vi "Measurement UI.vi"() -> ()   [LabVIEW 2020, in "Line Regulation.lvlib"]
uses:
  Line Regulation.lvlib
panel:
  out "Test Results.Input Voltage in V":dbl[](array[numeric])
  out "Output Voltage in V":dbl[](array[numeric])
  in  "Load SMU":refnum<k15>="DPS_4145_1/3"
  in  "Load DMM":refnum<k15>="DMM2"
  in  "Input DMM":refnum<k15>="DMM1"
  in  "Input SMU":refnum<k15>="DPS_4145_1/1"
  in  "Step":dbl=0.01
  in  "Stop":dbl=0.43
  in  "Start":dbl=0.03
  out "Line Regulation":cluster{"Iload (mA)":dbl[], "Vout (V)":dbl[]}(graph)
  out "Line Regulation (%)":dbl format="%#.3g"
  out "Line Regulation (%/V)":dbl format="%#.3g"
  in  "Nominal Output Voltage in V":dbl=3.3
  in  "Load Current in A":dbl=0.005
  # "Measurement Configurations"
  # "Measurement Results"
  # "Instruments"
  # "Input Voltage in V"
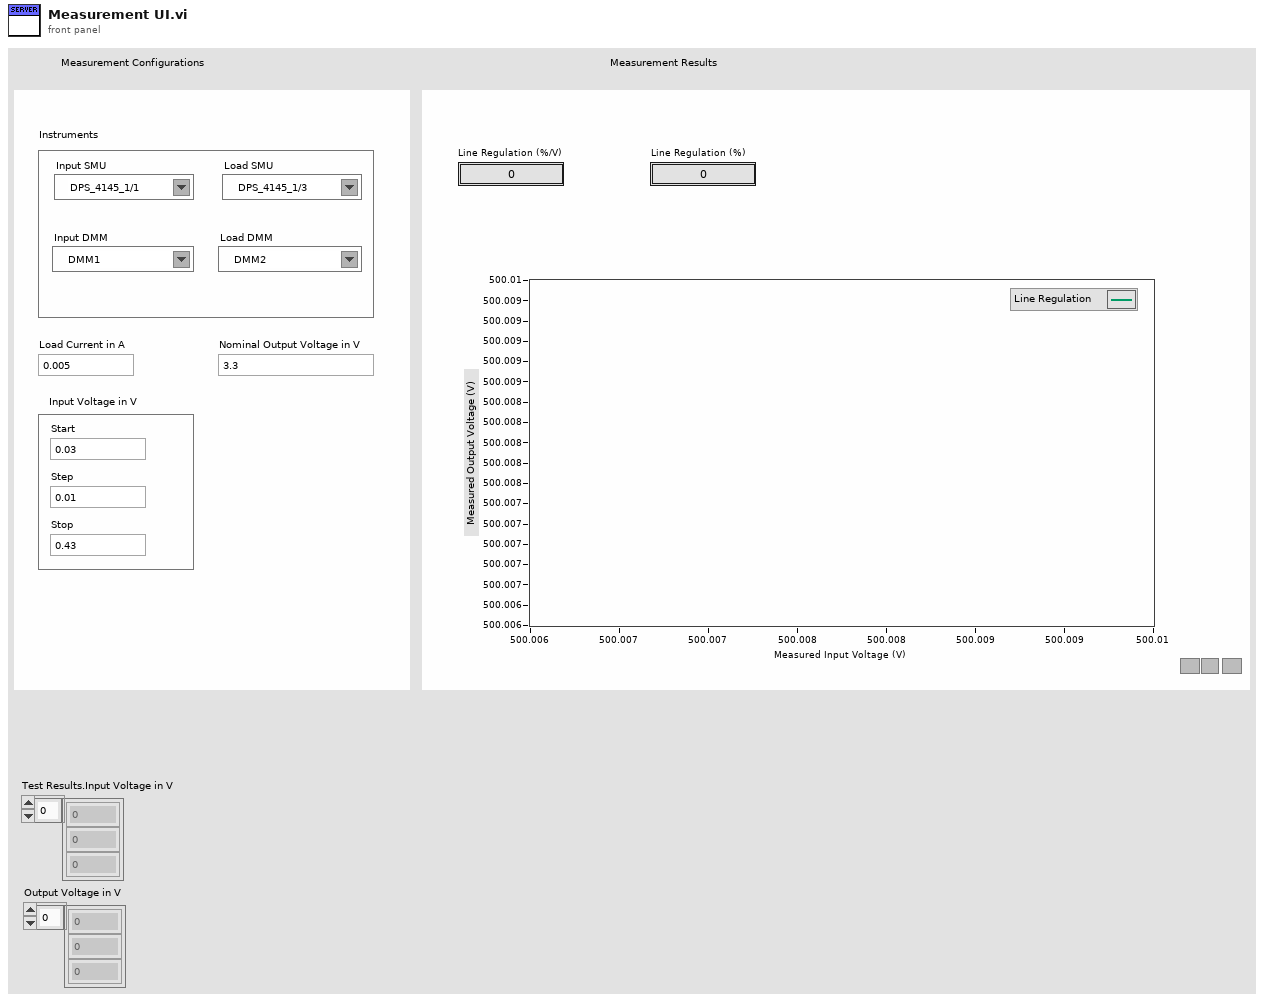
[diagram p1: front panel]
types:
  T1 = cluster{"Test Results.Input Voltage in V":dbl[], "Output Voltage in V":dbl[]}
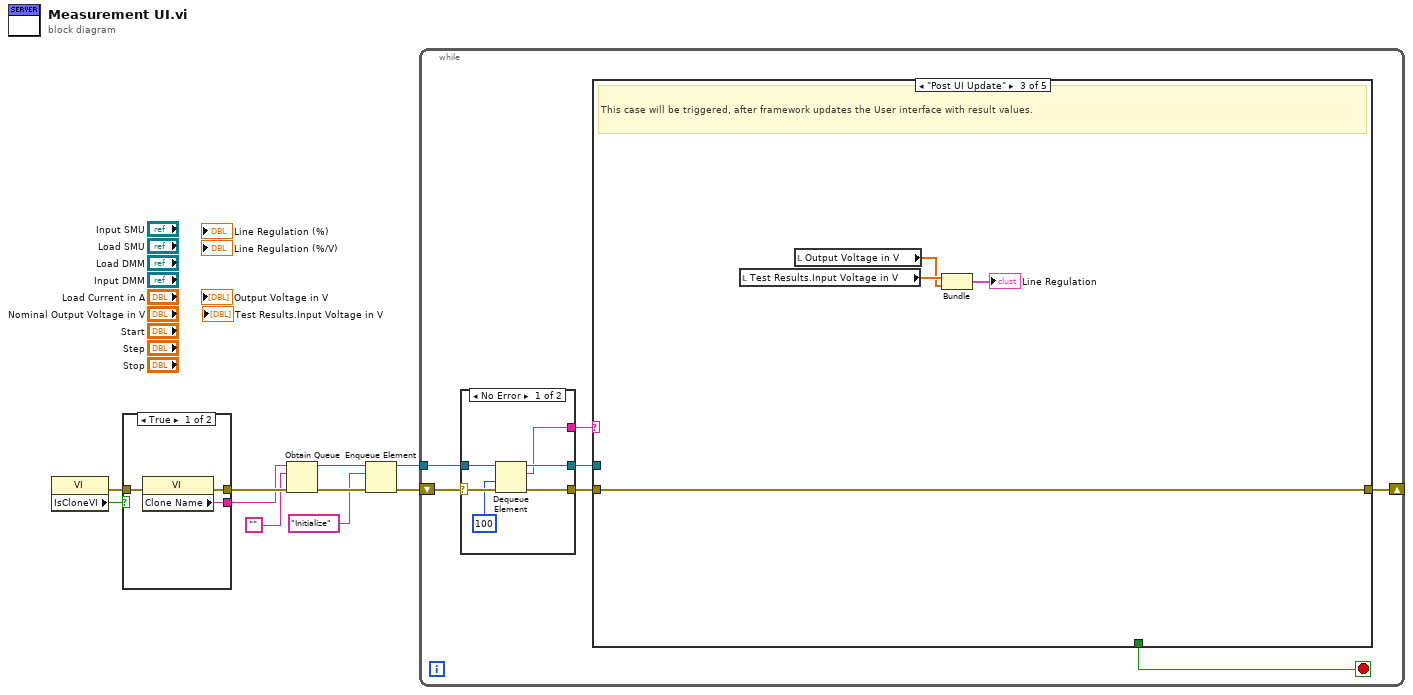
[diagram p0: block diagram]
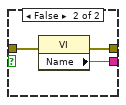
[diagram p2: hidden frame]
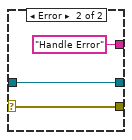
[diagram p3: hidden frame]
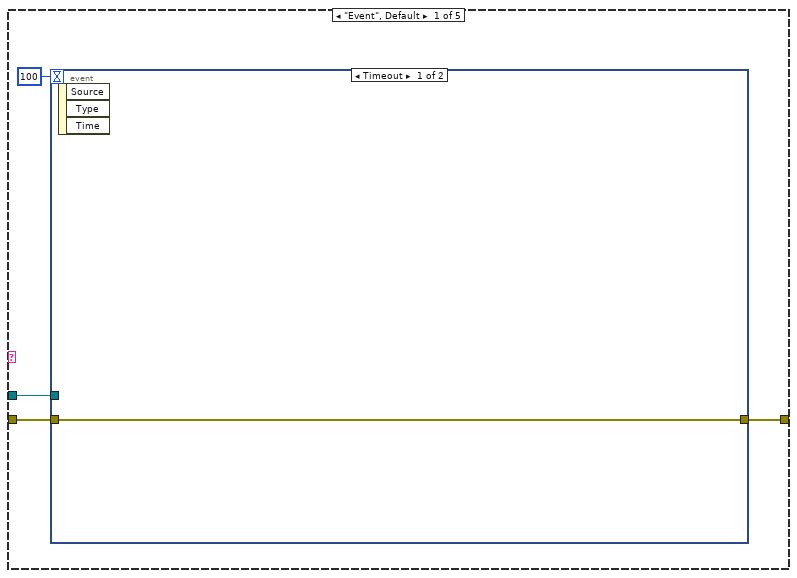
[diagram p4: hidden frame]
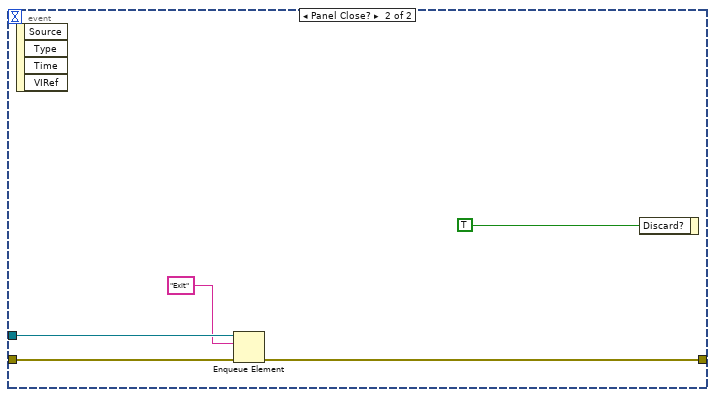
[diagram p5: hidden frame]
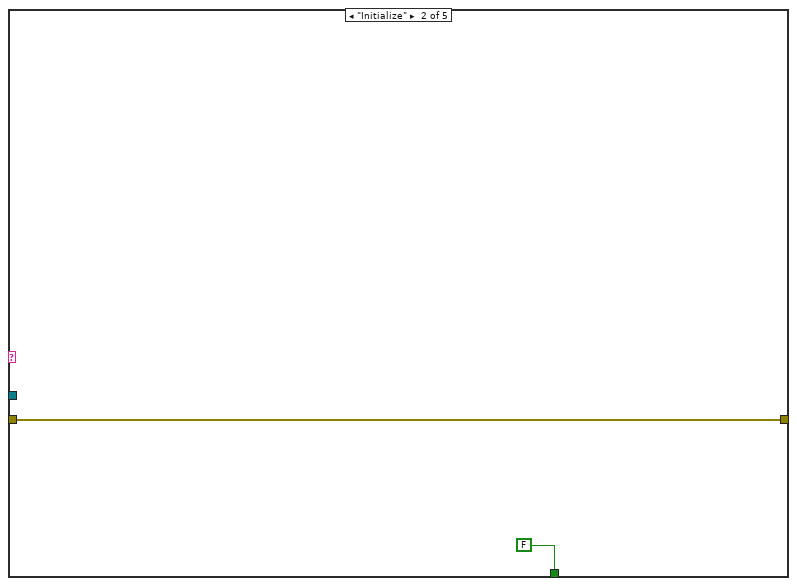
[diagram p6: hidden frame]
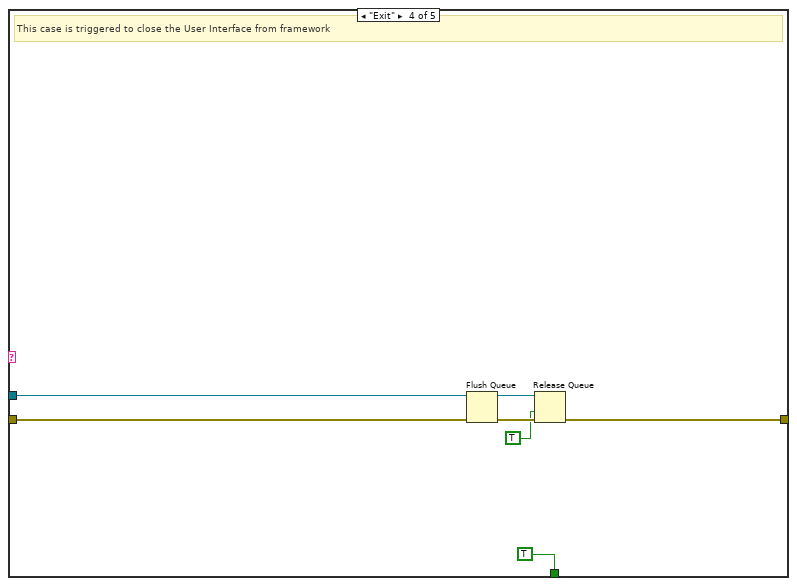
[diagram p7: hidden frame]
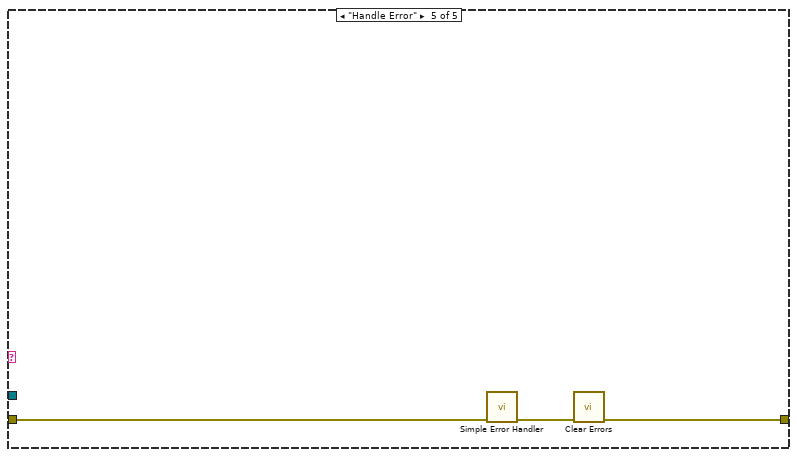
[diagram p8: hidden frame]
diagram:
  n1 = property class="VI"() -> (error out=w1:errorcluster, "IsCloneVI"=w2:bool)  [unwired: 2 in, 1 out]
  n2 = case shown="True" w2 {
    tunnel: [w13 w16] -> w10
    tunnel: [w12 w15] -> w9
    tunnel: w1 -> [w11 w14]
    frame True {
      n3 = property class="VI"(error in=w11) -> (error out=w13:errorcluster, "Clone Name"=w12:string)  [unwired: 1 in, 1 out]
    }
    frame False {
      n4 = property class="VI"(error in=w14) -> (error out=w16:errorcluster, "Name"=w15:string)  [unwired: 1 in, 1 out]
    }
  }
  n5 = Obtain Queue(name (unnamed)=w9, element data type="", error in (no error)=w10) -> (queue out=w6:refnum<queue>, error out=w8:errorcluster)  [unwired: 2 in, 1 out]
  n6 = Enqueue Element(queue=w6, element="Initialize", error in (no error)=w8) -> (queue out=w5:refnum<queue>, error out=w7:errorcluster)  [unwired: 1 in, 1 out]
  n7 = while {
    shift-right: [w18] -> _
    shift-left: w7 -> [w23]
    tunnel: w5 -> [w21]
    stop <- w17 stop-if-true
    n8 = case shown="No Error" w23 {
      selector: w23 -> [w29 w32]
      tunnel: [w28 w32] -> w22
      tunnel: w21 -> [w27 w31]
      tunnel: [w26 w31] -> w20
      tunnel: [w25 "Handle Error"] -> w19
      frame No Error {
        n9 = Dequeue Element(queue=w27, timeout in ms (-1)=100, error in (no error)=w29) -> (queue out=w26:refnum<queue>, element=w25:string, error out=w28:errorcluster)  [unwired: 1 out]
      }
      frame Error {
      }
    }
    n10 = case shown="\"Post UI Update\"" w19 {
      tunnel: w22 -> [w35 w44 w48 w55 w58]
      tunnel: w20 -> [w33 _ _ w53 _]
      tunnel: [w36 w44 w48 w50 w56] -> w18
      tunnel: [_ FALSE _ TRUE _] -> w17
      frame "Event", Default {
        n11 = event shown="[0] Timeout" {
          selector: _ -> [_ _]
          dyn-events: _ -> [_ _]
          timeout: 100 -> [_ _]
          tunnel: [w37 w40] -> w36
          tunnel: w35 -> [w37 w41]
          tunnel: w33 -> [_ w39]
          event Timeout {
            n12 = event-data() -> ()  [unwired: 1 in, 3 out]
          }
          event Panel Close? {
            n13 = event-data() -> ()  [unwired: 1 in, 4 out]
            n14 = Enqueue Element(queue=w39, element="Exit", error in (no error)=w41) -> (error out=w40:errorcluster)  [unwired: 1 in, 2 out]
            n15 = event-data("Discard?"=TRUE) -> ()  [unwired: 1 in, 1 out]
          }
        }
      }
      frame "Initialize" {
      }
      frame "Post UI Update" {
        # "This case will be triggered, after framework updates the User interface with result values."
        n16 = local read "Test Results.Input Voltage in V"() -> (w47:dbl[])
        n17 = local read "Output Voltage in V"() -> (w46:dbl[])
        n18 = Bundle("Test Results.Input Voltage in V"=w47, "Output Voltage in V"=w46) -> (→"Line Regulation":T1)  [unwired: 1 in]
      }
      frame "Exit" {
        # "This case is triggered to close the User Interface from framework"
        n19 = Flush Queue(queue=w53, error in (no error)=w55) -> (queue out=w52:refnum<queue>, error out=w51:errorcluster)  [unwired: 1 out]
        n20 = Release Queue(queue=w52, force destroy? (F)=TRUE, error in (no error)=w51) -> (error out=w50:errorcluster)  [unwired: 2 out]
      }
      frame "Handle Error" {
        n21 = call <vilib>:"Simple Error Handler.vi"("error in (no error)"=w58) -> ("error out"=w57:errorcluster)  [unwired: 4 in, 4 out]
        n22 = call <vilib>:"Clear Errors.vi"("error in (no error)"=w57) -> ("error out"=w56:errorcluster)  [unwired: 5 in, 1 out]
      }
    }
  }
